vi "Create All Message Queues.vi"(8 "error in (no error)":errorcluster, 10 "Master Queue In":refnum<queue>) -> (0 "error out":errorcluster, 3 "Message Queues out":T1)   [LabVIEW 2014, in "MeasurementControl Message Queue.lvlib"]
doc: "This VI creates and initializes all the message queues for your application. If your application requires more than one message queue, right-click the \"Message Queues\" constant above and select Open Type Def. Add the new Message Queue(s) to the type definition, then initialize them in this VI."
uses:
  MeasurementControl Message Queue.lvlib
  All Message Queues.ctl
  Message Cluster.ctl
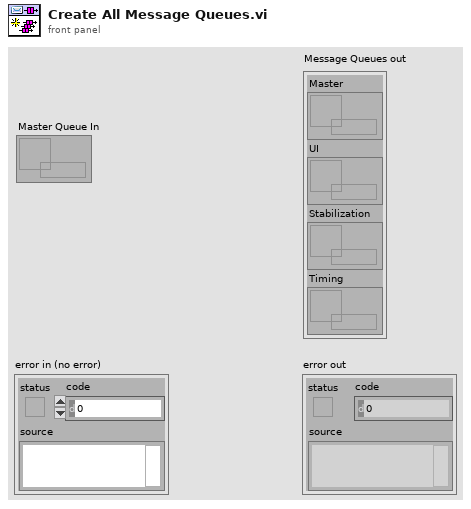
[diagram p1: front panel]
types:
  T1 = typedef "MeasurementControl Message Queue.lvlib/All Message Queues.ctl" = cluster{"Master":refnum<queue>, "UI":refnum<queue>, "Stabilization":refnum<queue>, "Timing":refnum<queue>}
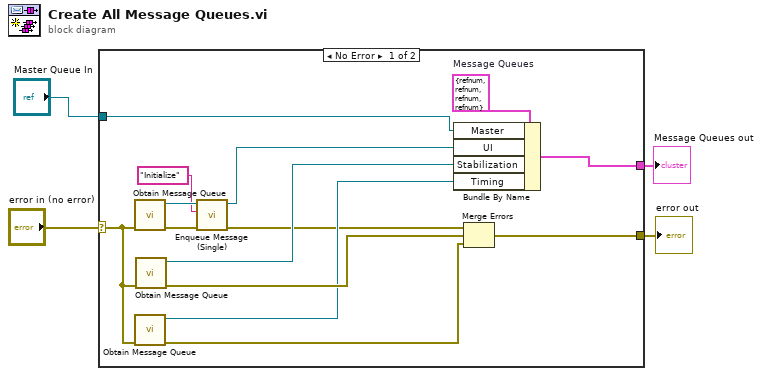
[diagram p0: block diagram]
diagram:
  n1 = case shown="No Error" "error in (no error)" {
    selector: "error in (no error)" -> [w10 w19]
    tunnel: [w16 w19] -> w4
    tunnel: [w17 _] -> w3
    tunnel: "Master Queue In" -> [w15 _]
    frame No Error {
      w18 = T1 {"Master"=refnum, "UI"=refnum, "Stabilization"=refnum, "Timing"=refnum}  # Message Queues
      n2 = call "Obtain Message Queue.vi"("error in (no error)"=w10) -> ("error out"=w8:errorcluster, "Message Queue"=w9:refnum<queue>)  [unwired: 9 in]
      n3 = call "Obtain Message Queue.vi"("error in (no error)"=w10) -> ("error out"=w11:errorcluster, "Message Queue"=w12:refnum<queue>)  [unwired: 9 in]
      n4 = call "Obtain Message Queue.vi"("error in (no error)"=w10) -> ("error out"=w13:errorcluster, "Message Queue"=w14:refnum<queue>)  [unwired: 9 in]
      n5 = call "Enqueue Message (Single).vi"("error in (no error)"=w8, "Message"="Initialize", "Message Queue"=w9) -> ("error out"=w7:errorcluster, "dup Message Queue"=w6:refnum<queue>)  [unwired: 7 in]
      n6 = Bundle By Name(cluster=w18, "Master"=w15, "UI"=w6, "Stabilization"=w14, "Timing"=w12) -> (w17:T1)
      n7 = Merge Errors(w7, w13, w11) -> (w16:errorcluster)
    }
    frame Error {
    }
  }
  "Message Queues out" <- w3
  "error out" <- w4
